vi "Sub Routing program.vi"(7 "FeedBack Channel":string[](array[string]), 8 "error in (no error)":errorcluster, 9 "Feature Step Enable":T1(array[cluster]), 11 "queue Out in":refnum<queue>) -> (0 "error out":errorcluster, 2 "Error Message":string, 3 "Queue out":refnum<queue>)   [LabVIEW 2015]
uses:
  Test  enqueue/AutoTest seq.ctl
  Galobal variable_TI.vi
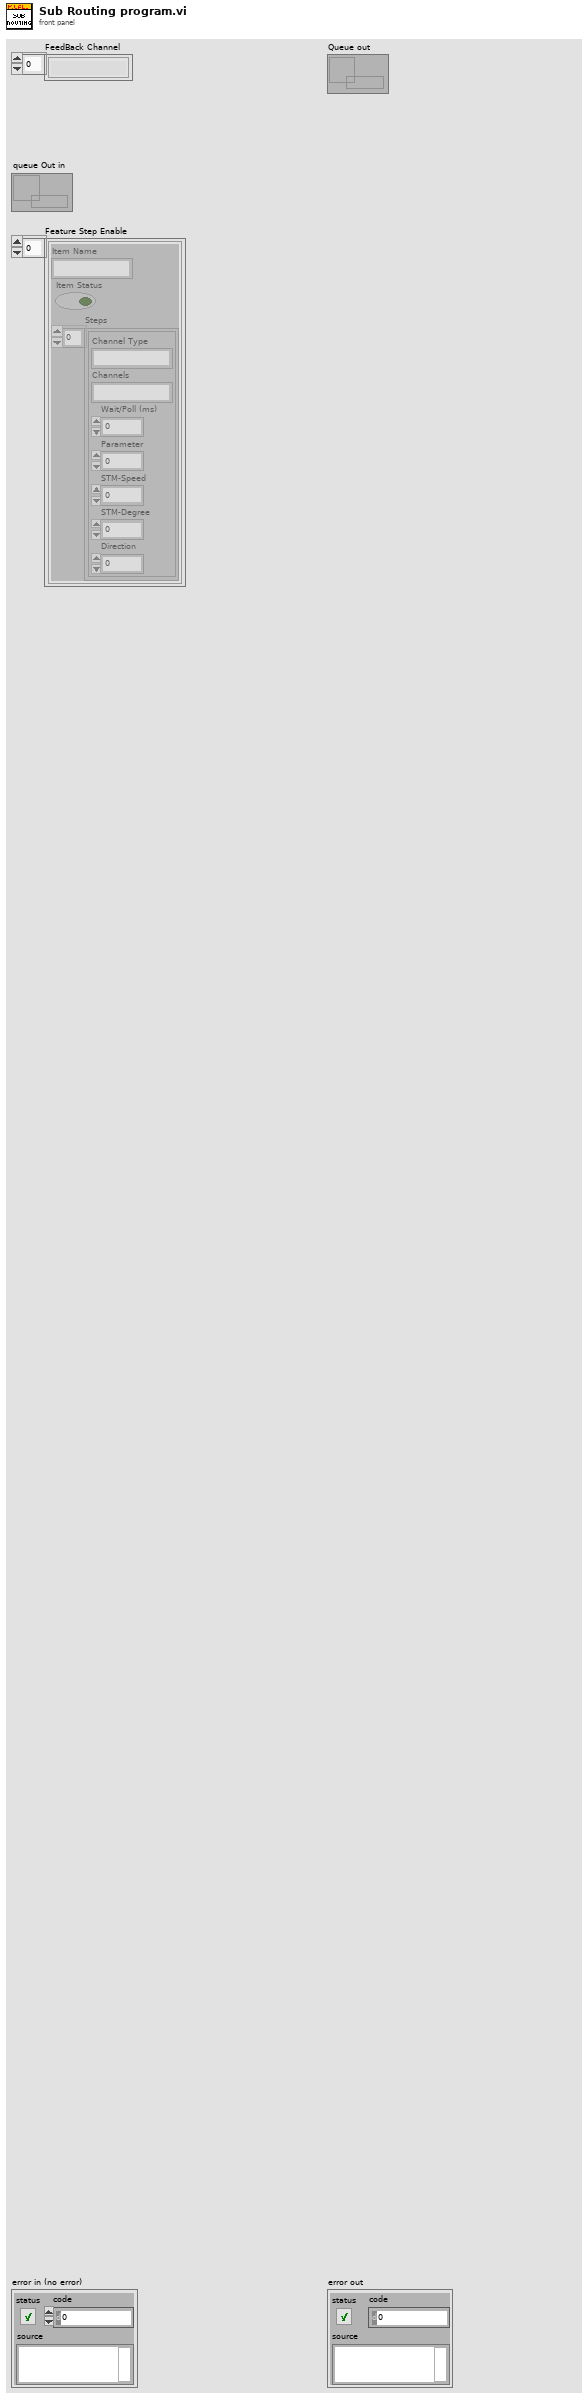
[diagram p1: front panel]
types:
  T1 = cluster{"Item Name":string, "Item Status":bool, "Steps":cluster{"Channel Type":string, "Channels":string, "Wait/Poll (ms)":u32, "Parameter":u8, "STM-Speed":i32, "STM-Degree":u32, "Direction":u8}[]}[]
  T2 = cluster{"Channel Type":string, "Channels":string, "Wait/Poll (ms)":u32, "Parameter":u8, "STM-Speed":i32, "STM-Degree":u32, "Direction":u8}[]
  T3 = cluster{"Emergency":bool, "Air Pressure":bool, "Saftey Sensor":bool, "Slide Servo  fault":bool, "LCD Pressing  Servo  fault":bool}
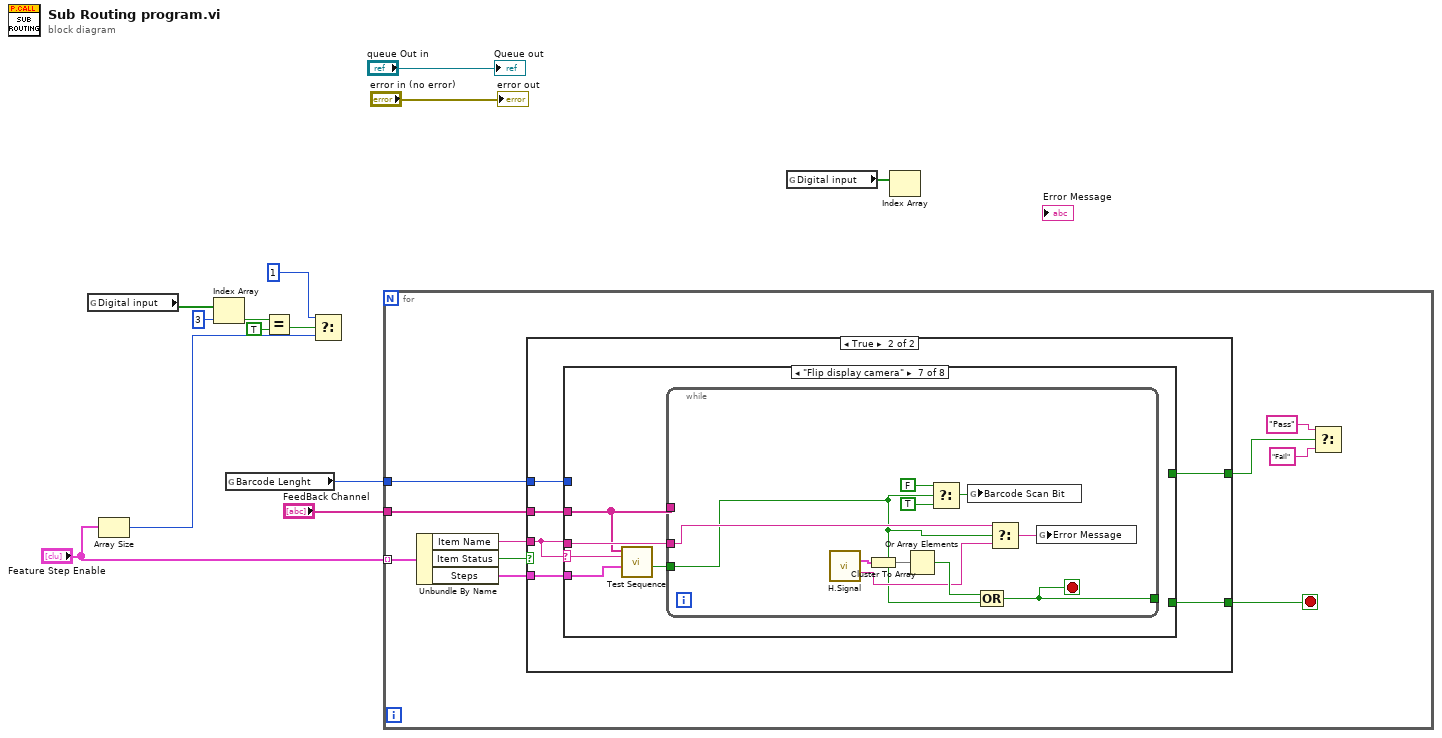
[diagram p0: block diagram]
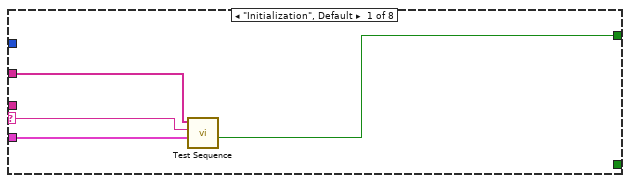
[diagram p3: hidden frame]
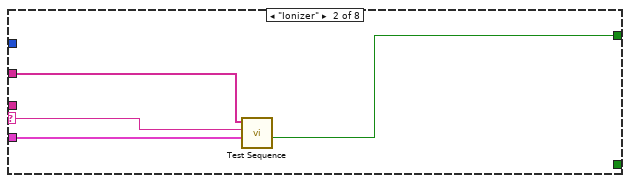
[diagram p4: hidden frame]
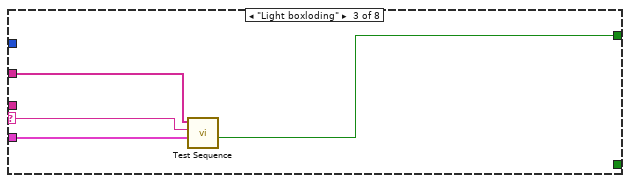
[diagram p5: hidden frame]
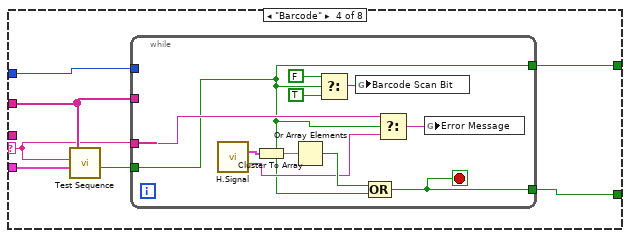
[diagram p6: hidden frame]
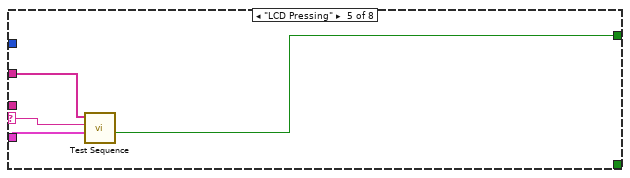
[diagram p7: hidden frame]
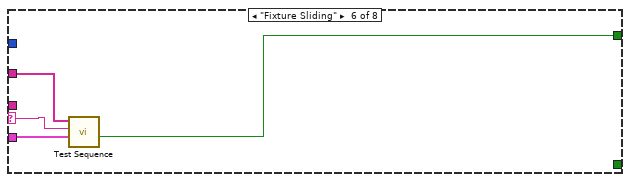
[diagram p8: hidden frame]
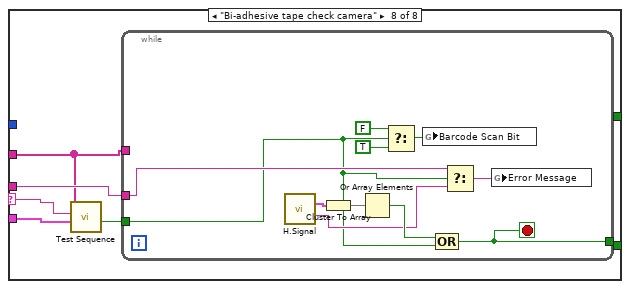
[diagram p9: hidden frame]
diagram:
  n1 = global read "Galobal variable_TI.vi" "Digital input"() -> (w10:bool[])
  n2 = Array Size(array="Feature Step Enable") -> (size(s)=w3:i32)
  n3 = Index Array(array=w10, index=3) -> (element=w9:bool)
  n4 = global read "Galobal variable_TI.vi" "Barcode Lenght"() -> (w11:i32)
  n5 = Equal?(x=w9, y=TRUE) -> (x = y?=w6:bool)
  n6 = Select(t=1, s=w6, f=w3) -> ()  [unwired: 1 out]
  n7 = for {
    tunnel: "Feature Step Enable" -> [w22] mode=indexing
    tunnel: "FeedBack Channel" -> [w23]
    tunnel: w11 -> [w18]
    stop <- w17 stop-if-true
    n8 = Unbundle By Name(w22) -> ("Item Name"=w20:string, "Item Status"=w19:bool, "Steps"=w21:T2)
    n9 = case shown="True" w19 {
      tunnel: w23 -> [_ w29]
      tunnel: w21 -> [_ w28]
      tunnel: w20 -> [_ w25]
      tunnel: w18 -> [_ w27]
      tunnel: [_ w26] -> w17
      tunnel: [_ w24] -> w14
      frame False {
      }
      frame True {
        n10 = case shown="\"Flip display camera\"" w25 {
          selector: w25 -> [w33 w36 w40 w45 w62 w66 w70 w86]
          tunnel: w29 -> [w31 w37 w41 w46 w61 w67 w71 w85]
          tunnel: w28 -> [w32 w35 w39 w44 w63 w65 w69 w87]
          tunnel: w27 -> [_ _ _ w48 _ _ _ _]
          tunnel: [_ _ _ w47 _ _ _ _] -> w26
          tunnel: w25 -> [_ _ _ _ _ _ w72 w88]
          tunnel: [w30 w34 w38 w42 w60 w64 _ _] -> w24
          frame "Initialization", Default {
            n11 = call "Test Sequence.vi"("FeedBack Channel"=w31, "Test Name"=w33, "Steps"=w32) -> ("Condition"=w30:bool)  [unwired: 4 in, 2 out]
          }
          frame "Ionizer" {
            n12 = call "Test Sequence.vi"("FeedBack Channel"=w37, "Test Name"=w36, "Steps"=w35) -> ("Condition"=w34:bool)  [unwired: 4 in, 2 out]
          }
          frame "Light boxloding" {
            n13 = call "Test Sequence.vi"("FeedBack Channel"=w41, "Test Name"=w40, "Steps"=w39) -> ("Condition"=w38:bool)  [unwired: 4 in, 2 out]
          }
          frame "Barcode" {
            n14 = call "Test Sequence.vi"("FeedBack Channel"=w46, "Test Name"=w45, "Steps"=w44) -> ("Condition"=w43:bool)  [unwired: 4 in, 2 out]
            n15 = while {
              tunnel: w46 -> [_]
              tunnel: w45 -> [w52]
              tunnel: w48 -> [_]
              tunnel: [w53] -> w47
              tunnel: w43 -> [w49]
              tunnel: [w49] -> w42
              stop <- w53 stop-if-true
              n16 = call "H.Signal.vi"() -> ("H.Signal"=w59:T3, "Error Message"=w51:string)  [unwired: 11 in, 3 out]
              n17 = Cluster To Array(cluster=w59) -> (array=w58:bool[])
              n18 = Or Array Elements(Boolean array=w58) -> (logical OR=w57:bool)
              n19 = Select(t=FALSE, s=w49, f=TRUE) -> (s? t:f=w55:bool)
              n20 = global write "Galobal variable_TI.vi" "Barcode Scan Bit"(w55) -> ()
              n21 = Compound Arithmetic op=OR(w57, w49) -> (w53:bool)
              n22 = Select(t=w52, s=w49, f=w51) -> (s? t:f=w50:string)
              n23 = global write "Galobal variable_TI.vi" "Error Message"(w50) -> ()
            }
          }
          frame "LCD Pressing" {
            n24 = call "Test Sequence.vi"("FeedBack Channel"=w61, "Test Name"=w62, "Steps"=w63) -> ("Condition"=w60:bool)  [unwired: 4 in, 2 out]
          }
          frame "Fixture Sliding" {
            n25 = call "Test Sequence.vi"("FeedBack Channel"=w67, "Test Name"=w66, "Steps"=w65) -> ("Condition"=w64:bool)  [unwired: 4 in, 2 out]
          }
          frame "Flip display camera" {
            n26 = call "Test Sequence.vi"("FeedBack Channel"=w71, "Test Name"=w70, "Steps"=w69) -> ("Condition"=w68:bool)  [unwired: 4 in, 2 out]
            n27 = while {
              tunnel: w71 -> [_]
              tunnel: w72 -> [w76]
              tunnel: [w77] -> _
              tunnel: w68 -> [w73]
              stop <- w77 stop-if-true
              n28 = call "H.Signal.vi"() -> ("H.Signal"=w83:T3, "Error Message"=w75:string)  [unwired: 11 in, 3 out]
              n29 = Cluster To Array(cluster=w83) -> (array=w82:bool[])
              n30 = Or Array Elements(Boolean array=w82) -> (logical OR=w81:bool)
              n31 = Select(t=FALSE, s=w73, f=TRUE) -> (s? t:f=w79:bool)
              n32 = global write "Galobal variable_TI.vi" "Barcode Scan Bit"(w79) -> ()
              n33 = Compound Arithmetic op=OR(w81, w73) -> (w77:bool)
              n34 = Select(t=w76, s=w73, f=w75) -> (s? t:f=w74:string)
              n35 = global write "Galobal variable_TI.vi" "Error Message"(w74) -> ()
            }
          }
          frame "Bi-adhesive tape check camera" {
            n36 = call "Test Sequence.vi"("FeedBack Channel"=w85, "Test Name"=w86, "Steps"=w87) -> ("Condition"=w84:bool)  [unwired: 4 in, 2 out]
            n37 = while {
              tunnel: w85 -> [_]
              tunnel: w88 -> [w92]
              tunnel: [w93] -> _
              tunnel: w84 -> [w89]
              stop <- w93 stop-if-true
              n38 = call "H.Signal.vi"() -> ("H.Signal"=w99:T3, "Error Message"=w91:string)  [unwired: 11 in, 3 out]
              n39 = Cluster To Array(cluster=w99) -> (array=w98:bool[])
              n40 = Or Array Elements(Boolean array=w98) -> (logical OR=w97:bool)
              n41 = Select(t=FALSE, s=w89, f=TRUE) -> (s? t:f=w95:bool)
              n42 = global write "Galobal variable_TI.vi" "Barcode Scan Bit"(w95) -> ()
              n43 = Compound Arithmetic op=OR(w97, w89) -> (w93:bool)
              n44 = Select(t=w92, s=w89, f=w91) -> (s? t:f=w90:string)
              n45 = global write "Galobal variable_TI.vi" "Error Message"(w90) -> ()
            }
          }
        }
      }
    }
    n46 = Select(t="Pass", s=w14, f="Fail") -> ()  [unwired: 1 out]
  }
  n47 = global read "Galobal variable_TI.vi" "Digital input"() -> (w12:bool[])
  n48 = Index Array(array=w12) -> ()  [unwired: 1 in, 1 out]
  "error out" <- "error in (no error)"
  "Queue out" <- "queue Out in"
